vi "Inline Wheel State.vi"(8 "Allowable Variation from Ideal":dbl, 9 "Ideal Slip Percent":dbl, 10 "Chassis Speed":dbl, 11 "Wheel Speed":dbl) -> (1 "Error":dbl, 2 "Inline Slip":bool)   [LabVIEW 2013]
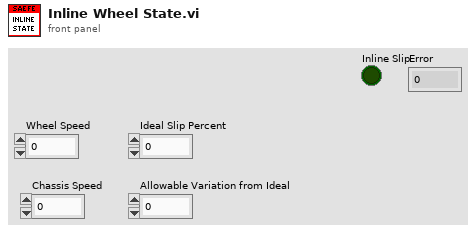
[diagram p1: front panel]
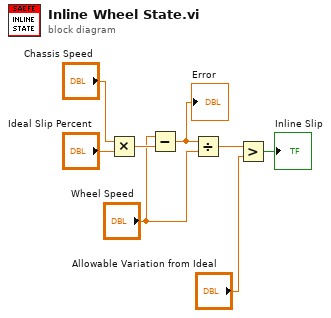
[diagram p0: block diagram]
diagram:
  n1 = Multiply(x="Chassis Speed", y="Ideal Slip Percent") -> (x*y=w6:dbl)
  n2 = Subtract(x="Wheel Speed", y=w6) -> (x-y=w5:dbl)
  "Error" <- w5
  n3 = Divide(x=w5, y="Wheel Speed") -> (x/y=w3:dbl)
  n4 = Greater?(x=w3, y="Allowable Variation from Ideal") -> (0:→"Inline Slip":bool)
